vi "Warranty Gas Rack Main (FPGA).vi"() -> ()   [LabVIEW 2013]
uses:
  TypeDef/FPGADataCluster.ctl
  <vilib>/Platform/TimedLoop/XDataNode/timing_clust.ctl
  <vilib>/Platform/TimedLoop/XDataNode/nitl_modes.ctl
  <vilib>/Platform/TimedLoop/XDataNode/wakeup.ctl
  <vilib>/rvi/FXPMathLib/basic elements/FxpIntAccumulator/subVIs/nifxpmath_IntAccumulator_SimConfig.ctl
  <vilib>/rvi/FXPMathLib/FxpSqrt/subVIs/nifxpmath_Sqrt_SimConfig.ctl
  <vilib>/fxp/LVFixedPointOverflowPolicyTypeDef.ctl
  <vilib>/rvi/Emulation/niFpgaSctlEmulationGetInTimedLoop.vi
  <vilib>/rvi/Emulation/niFpgaEmulationReportErrorSimple.vi
  <vilib>/rvi/Emulation/niFpgaGetClockAttributes.vi
  <vilib>/rvi/eio/common/nirviEmuTemplateMethod_errors.vi
  <vilib>/rvi/Analysis/common/codeGenErrors/XNode/niFpgaXNodeCodeGenErrorHandle.vi
  <vilib>/rvi/Emulation/niFpgaCriticalErrorInLSC.vi
  <vilib>/rvi/FXPMathLib/basic elements/FxpIntAccumulator/simVIs/DllFxpIntAccumulator_sub.vi
  <vilib>/rvi/interface/RandomDataEmulation/nirviRandomDataFPGAFIFO.vi
  <vilib>/rvi/interface/RandomDataEmulation/niFpgaRandomDataHandleErrors.vi
  <vilib>/rvi/FXPMathLib/FxpSqrt/simVIs/DllSqrtTemp_sub.vi
  <vilib>/rvi/FXPMathLib/FxpSub/XNode/nifxpmath_Sub.xnode
  <vilib>/eio/EIONode/EIONode.xnode
  <vilib>/rvi/Analysis/measure/mean-var-std/XNode/niFpgaMean-Var-Std.xnode
  <vilib>/Platform/TimedLoop/XDataNode/XDataNode.xnode
  <vilib>/rvi/FXPMathLib/basic elements/FxpIntAccumulator/XNode/nifxpmath_IntAccumulator.xnode
  <vilib>/rvi/FXPMathLib/FxpMul/XNode/nifxpmath_Multiplier.xnode
  <vilib>/rvi/DataTransferAndStorage/Container/XNode/niFpgaContainer.xnode
  <vilib>/rvi/interface/RandomDataEmulation/nirviRandomDataFpgaReadWriteTemplate.vi
  <vilib>/rvi/Analysis/measure/butterworth/XNode/niFpgaButterworthFilter.xnode
  <vilib>/rvi/Analysis/measure/dc-rms/XNode/niFpgaDC-RMS.xnode
  <vilib>/rvi/FXPMathLib/FxpSqrt/XNode/nifxpmath_Sqrt.xnode
  <vilib>/Platform/TimedLoop/XDataNode/XDNodeRunTimeDep.lvlib
  <vilib>/rvi/FXPMathLib/sim/FxpSim.dll
panel:
  out "Version":u8=1
  in  "NeedleValve":bool
  in  "CtCuttoff":fxp<+,24,5>
  in  "Brushed Speed":bool
  in  "StableTrigger":fxp<+/-,20,5>
  in  "Count 2(uS)":u32=20
  out "AI3":fxp<+/-,24,5>
  out "AI7":fxp<+/-,24,5>
  out "AI6":fxp<+/-,24,5>
  out "AI4":fxp<+/-,24,5>
  out "AI2":fxp<+/-,24,5>
  out "AI1":fxp<+/-,24,5>
  out "AI0":fxp<+/-,24,5>
  out "Actual Loop Time 2":u32
  out "Actual Loop Time":u32
  in  "Count 1(uS)":u32=100
  in  "Hysteresis":fxp<+,24,5>
  out "DataCluster":T1 {"Speed" format="%#_6f"; "Controller Voltage" format="%#_6f"; "Controller Current" format="%#_6f"; "Temperature" format="%#_6f"}
  in  "PWM Period (ticks)":u32
  in  "PWM Duty":i32
  in  "Deadhead":bool
  in  "PSenable":bool
  in  "PresCtrl":fxp<+/-,20,5>
  in  "VoltCtrl":fxp<+/-,20,5>
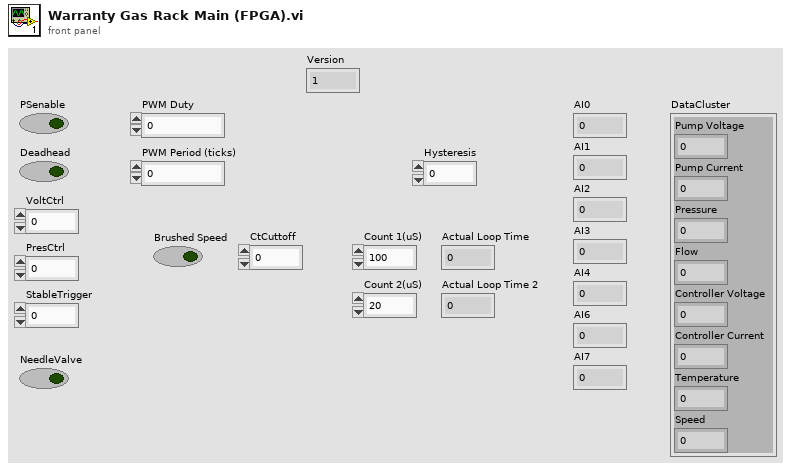
[diagram p1: front panel]
types:
  T1 = typedef "FPGADataCluster.ctl" = cluster{"Pump Voltage":fxp<+/-,25,15>, "Pump Current":fxp<+/-,25,15>, "Pressure":fxp<+/-,25,15>, "Flow":fxp<+/-,25,15>, "Controller Voltage":fxp<+/-,25,15>, "Controller Current":fxp<+/-,25,15>, "Temperature":fxp<+/-,25,15>, "Speed":fxp<+/-,25,15>}
  T2 = typedef "XDNodeRunTimeDep.lvlib/timing_clust.ctl" = cluster{"Expected End [f-1]":u64, "Actual End [f-1]":u64, "Finished Late? [f-1]":bool, "Expected End [i-1]":u64, "Actual End [i-1]":u64, "Finished Late? [i-1]":bool, "Expected Start [i]":u64, "Actual Start [i]":u64, "Expected Start [f]":u64, "Actual Start [f]":u64, "Source Name":string, "Structure Name":string, "Period":i64, "Deadline":i64, "Offset":i64, "Start":i64, "Priority":i32, "Timeout":i32, "Mode":T3, "Wakeup Reason":T4, "Error":errorcluster, "Source Type":string, "Secondary Source Type":string, "Global End Time":u64, "Global Start Time":u64, "Frame Duration":u64, "Iteration Duration":u64, "Assigned CPU":i32, "I/O Scan Engine Mode":u32}
  T3 = typedef "XDNodeRunTimeDep.lvlib/nitl_modes.ctl" = enum32{"No Change", "Process missed periods, maintain original phase", "Discard missed periods, maintain original phase", "Process missed periods, ignore original phase", "Discard missed periods, ignore original phase"}
  T4 = typedef "XDNodeRunTimeDep.lvlib/wakeup.ctl" = enum32{"Normal", "Aborted", "Asynchronous wakeup", "Timing source error", "Timed loop error", "Timeout"}
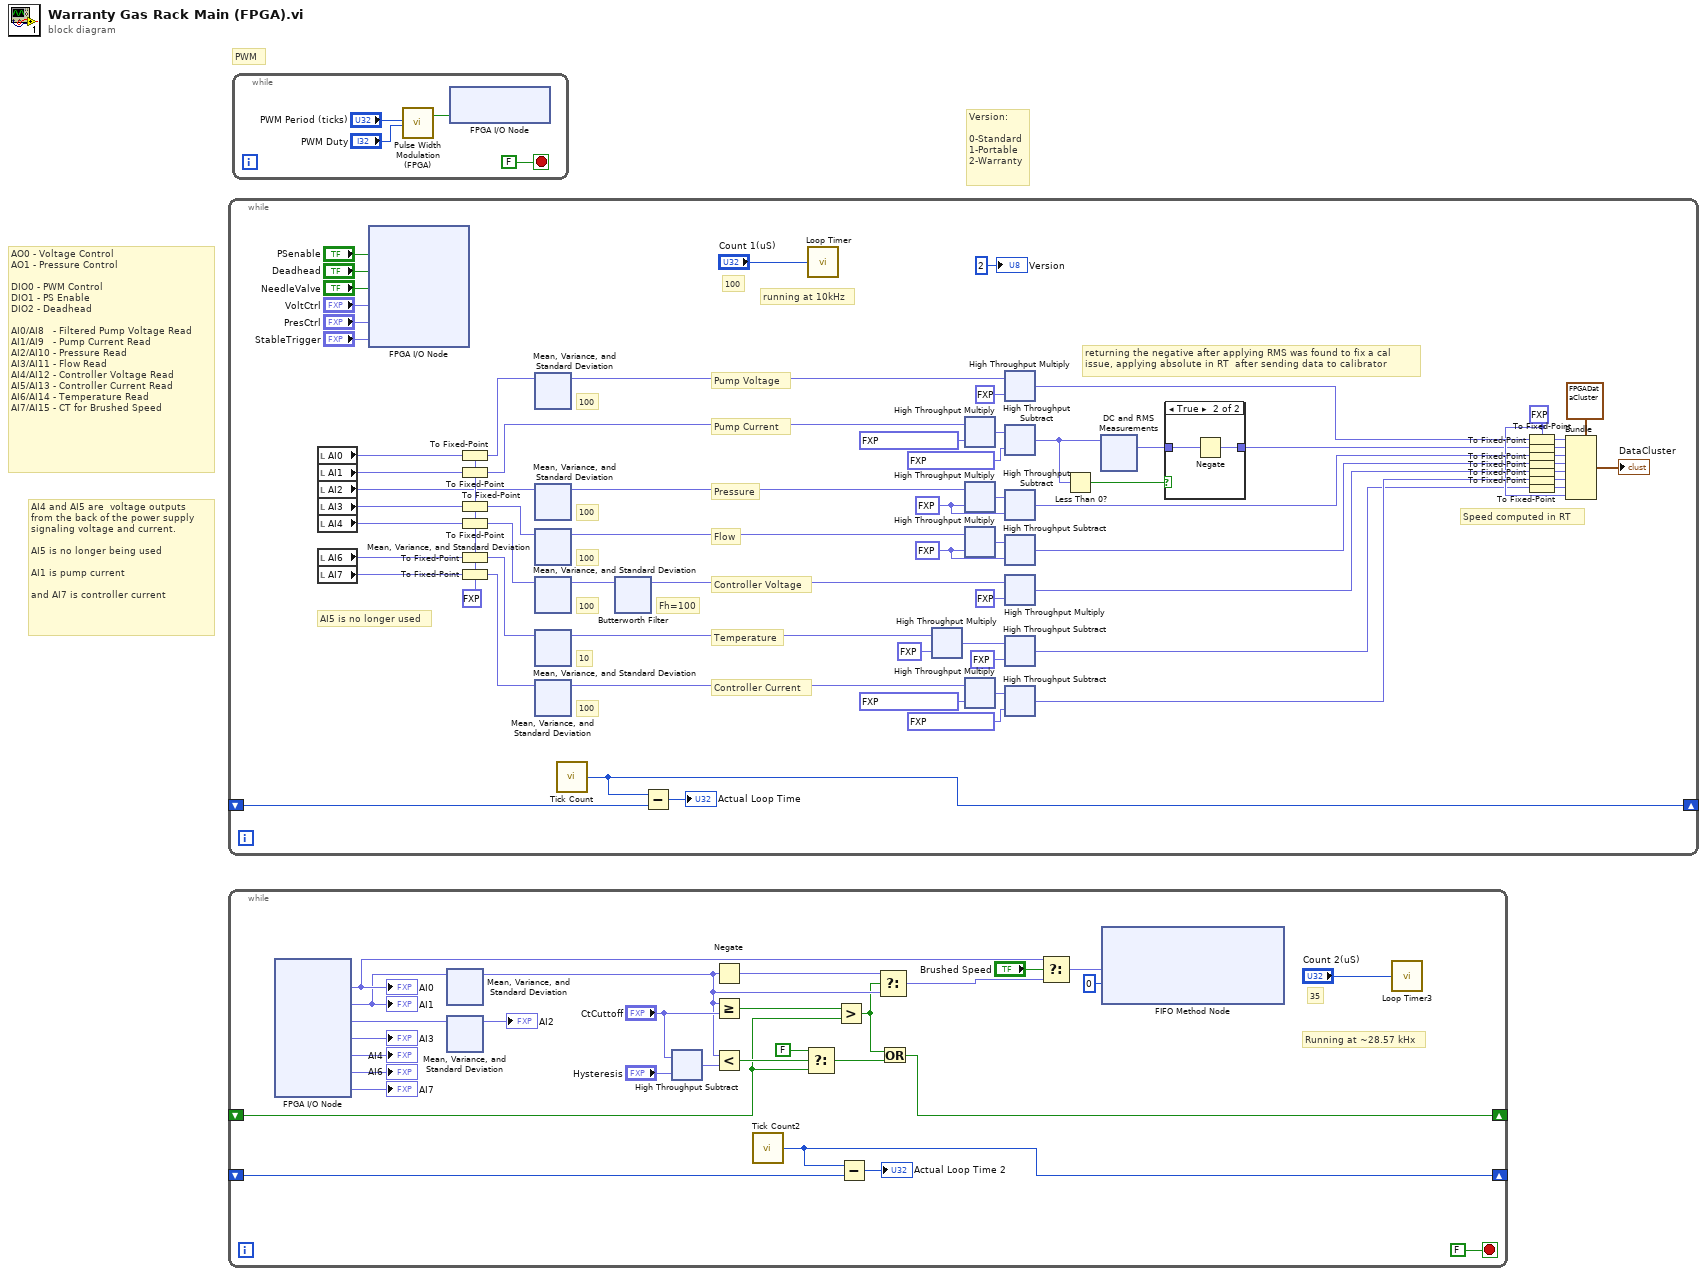
[diagram p0: block diagram]
diagram:
  # "Version:\n\n0-Standard\n1-Portable\n2-Warranty"
  # "PWM"
  # "AI4 and AI5 are  voltage outputs\nfrom the back of the power supply\nsignaling voltage and current.\n\nAI5 is no longer being used\n\nAI1 is pump current\n\nand AI7 is controller current"
  # "AO0 - Voltage Control\nAO1 - Pressure Control\n\nDIO0 - PWM Control\nDIO1 - PS Enable\nDIO2 - Deadhead\n\nAI0/AI8   - Filtered Pump Voltage Read\nAI1/AI9   - Pump Current Read\nAI2/AI10 - Pressure Read\nAI3/AI11 - Flow Read\nAI4/AI12 - Controller Voltage Read\nAI5/AI13 - Controller Current Read\nAI6/AI14 - Temperature Read\nAI7/AI15 - CT for Brushed Speed"
  n1 = while {
    shift-right: [w33] -> _
    shift-left: _ -> [w32]
    stop <- FALSE stop-if-true
    w20 = fxp<+,9,9> 258.0 ("y")
    w43 = fxp<+,24,5> 0.0 ("AI4")
    w11 = fxp<+/-,25,15> 0.0 ("Element")
    w4 = fxp<+,8,8> 170.0 ("y")
    # "Fh=100"
    # "10"
    # "100"
    # "100"
    # "100"
    # "100"
    # "100"
    # "Temperature"
    # "Controller Current"
    # "Controller Voltage"
    # "Flow"
    # "Pressure"
    # "Pump Current"
    # "Pump Voltage"
    # "100"
    # "Speed computed in RT"
    # "returning the negative after applying RMS was found to fix a cal\nissue, applying absolute in RT  after sending data to calibrator"
    # "AI5 is no longer used"
    # "running at 10kHz"
    n2 = local read "AI0"() -> (w31:fxp<+/-,24,5>)
    n3 = local read "AI1"() -> (w30:fxp<+/-,24,5>)
    n4 = local read "AI2"() -> (w15:fxp<+/-,24,5>)
    n5 = local read "AI3"() -> (w28:fxp<+/-,24,5>)
    n6 = local read "AI4"() -> (w27:fxp<+/-,24,5>)
    n7 = local read "AI6"() -> (w26:fxp<+/-,24,5>)
    n8 = local read "AI7"() -> (w29:fxp<+/-,24,5>)
    n9 = xnode "FPGA I/O Node"("RMC/DIO1"="PSenable", "RMC/DIO2"="Deadhead", "RMC/DIO3"="NeedleValve", "AO0"="VoltCtrl", "AO1"="PresCtrl", "AO2"="StableTrigger") -> ()  [unwired: 6 in, 6 out]
    n10 = To Fixed-Point(fixed-point type=w43, number=w31) -> (fixed-point=w36:fxp<+,24,5>)
    n11 = To Fixed-Point(fixed-point type=w43, number=w30) -> (fixed-point=w10:fxp<+,24,5>)
    n12 = To Fixed-Point(fixed-point type=w43, number=w28) -> (fixed-point=w42:fxp<+,24,5>)
    n13 = To Fixed-Point(fixed-point type=w43, number=w27) -> (fixed-point=w41:fxp<+,24,5>)
    n14 = To Fixed-Point(fixed-point type=w43, number=w26) -> (fixed-point=w35:fxp<+,24,5>)
    n15 = To Fixed-Point(fixed-point type=w43, number=w29) -> (fixed-point=w17:fxp<+,24,5>)
    n16 = xnode "Mean, Variance, and Standard Deviation"("input data"=w36) -> ("mean"=w40:fxp<+,24,5>)  [unwired: 1 in, 1 out]
    n17 = xnode "Mean, Variance, and Standard Deviation"("input data"=w15) -> ("mean"=w14:fxp<+/-,24,5>)  [unwired: 1 in, 1 out]
    n18 = xnode "Mean, Variance, and Standard Deviation"("input data"=w42) -> ("mean"=w39:fxp<+,24,5>)  [unwired: 1 in, 1 out]
    n19 = xnode "Mean, Variance, and Standard Deviation"("input data"=w41) -> ("mean"=w13:fxp<+,24,5>)  [unwired: 1 in, 1 out]
    n20 = xnode "Mean, Variance, and Standard Deviation"("input data"=w35) -> ("mean"=w7:fxp<+,24,5>)  [unwired: 1 in, 1 out]
    n21 = xnode "Mean, Variance, and Standard Deviation"("input data"=w17) -> ("mean"=w16:fxp<+,24,5>)  [unwired: 1 in, 1 out]
    n22 = call "Tick Count"() -> ("Tick Count(uSec)"=w33:u32)
    n23 = xnode "Butterworth Filter"("input data"=w13) -> ("output data"=w12:fxp<+/-,29,10>)  [unwired: 2 in]
    n24 = Subtract(x=w33, y=w32) -> (x-y=→"Actual Loop Time":u32)
    n25 = call "Loop Timer"("Count(uSec)"="Count 1(uS)") -> ()  [unwired: 1 out]
    n26 = xnode ("High Throughput Multiply")("x"=w7, "y"=fxp<+/-,9,9> 145.0) -> ("x*y"=w6:fxp<+/-,25,15>)
    n27 = xnode ("High Throughput Multiply")("x"=w10, "y"=fxp<+/-,20,7> 24.0384521484375 ("Volt")) -> ("x*y"=w66:fxp<+/-,44,12>)
    n28 = xnode ("High Throughput Multiply")("x"=w14, "y"=w20) -> ("x*y"=w22:fxp<+/-,33,14>)
    n29 = xnode ("High Throughput Multiply")("x"=w39, "y"=w4) -> ("x*y"=w5:fxp<+/-,25,15>)
    n30 = xnode ("High Throughput Multiply")("x"=w16, "y"=fxp<+/-,20,7> 24.0384521484375 ("Volt")) -> ("x*y"=w37:fxp<+/-,44,12>)
    n31 = xnode ("High Throughput Multiply")("x"=w40, "y"=fxp<+/-,24,5> 11.0) -> ("x*y"=w48:fxp<+/-,25,15>)
    n32 = xnode "High Throughput Subtract"("x"=w66, "y"=fxp<+/-,20,7> 60.09619140625 ("Volt")) -> ("x-y"=w19:fxp<+/-,25,15>)
    n33 = xnode "High Throughput Subtract"("x"=w22, "y"=w20) -> ("x-y"=w21:fxp<+/-,34,15>)
    n34 = xnode "High Throughput Subtract"("x"=w5, "y"=w4) -> ("x-y"=w3:fxp<+/-,26,16>)
    n35 = xnode ("High Throughput Multiply")("x"=w12, "y"=fxp<+,8,8> 11.0) -> ("x*y"=w47:fxp<+/-,25,15>)
    n36 = xnode "High Throughput Subtract"("x"=w6, "y"=fxp<+/-,8,8> 100.0) -> ("x-y"=w8:fxp<+/-,21,10>)
    n37 = xnode "High Throughput Subtract"("x"=w37, "y"=fxp<+/-,20,7> 60.09619140625 ("Volt")) -> ("x-y"=w18:fxp<+/-,25,15>)
    n38 = Less Than 0?(x=w19) -> (x < 0?=w24:bool)
    n39 = xnode "DC and RMS Measurements"("input data"=w19) -> ("RMS"=w23:fxp<+,25,15>)  [unwired: 1 in, 1 out]
    n40 = case shown="True" w24 {
      tunnel: w23 -> [w229 w231]
      tunnel: [w229 w230] -> w2
      frame False {
      }
      frame True {
        n41 = Negate(x=w231) -> (-x=w230:fxp<+/-,26,16>)
      }
    }
    n42 = To Fixed-Point(fixed-point type=w11, number=w48) -> (fixed-point=w55:fxp<+/-,25,15>)
    n43 = To Fixed-Point(fixed-point type=w11, number=w2) -> (fixed-point=w56:fxp<+/-,25,15>)
    n44 = To Fixed-Point(fixed-point type=w11, number=w21) -> (fixed-point=w57:fxp<+/-,25,15>)
    n45 = To Fixed-Point(fixed-point type=w11, number=w3) -> (fixed-point=w58:fxp<+/-,25,15>)
    n46 = To Fixed-Point(fixed-point type=w11, number=w47) -> (fixed-point=w59:fxp<+/-,25,15>)
    n47 = To Fixed-Point(fixed-point type=w11, number=w18) -> (fixed-point=w50:fxp<+/-,25,15>)
    n48 = To Fixed-Point(fixed-point type=w11, number=w8) -> (fixed-point=w51:fxp<+/-,25,15>)
    n49 = Bundle(cluster=T1 {"Pump Voltage"=0.0, "Pump Current"=0.0, "Pressure"=0.0, "Flow"=0.0, "Controller Voltage"=0.0, "Controller Current"=0.0, "Temperature"=0.0, "Speed"=0.0} ("DataCluster"), "Pump Voltage"=w55, "Pump Current"=w56, "Pressure"=w57, "Flow"=w58, "Controller Voltage"=w59, "Controller Current"=w50, "Temperature"=w51, "Speed"=w11) -> (→"DataCluster":T1)
    "Version" <- u8 2
  }
  n50 = while {
    shift-right: [w669] -> _
    shift-left: _ -> [w670]
    shift-right: [w646] -> _
    shift-left: _ -> [w650]
    stop <- FALSE stop-if-true
    # "Running at ~28.57 kHx"
    # "35"
    n51 = xnode "FPGA I/O Node"() -> ("AI0"=w659:fxp<+/-,24,5>, "AI1"=w657:fxp<+/-,24,5>, "AI2"=w645:fxp<+/-,24,5>, "AI3"=→"AI3":fxp<+/-,24,5>, "AI4"=→"AI4":fxp<+/-,24,5>, "AI6"=→"AI6":fxp<+/-,24,5>, "AI7"=→"AI7":fxp<+/-,24,5>)  [unwired: 7 in, 7 out]
    "AI0" <- w659
    "AI1" <- w657
    n52 = xnode "Mean, Variance, and Standard Deviation"("input data"=w657) -> ("mean"=w653:fxp<+/-,24,5>)  [unwired: 1 in, 1 out]
    n53 = xnode "Mean, Variance, and Standard Deviation"("input data"=w645) -> ("mean"=→"AI2":fxp<+/-,24,5>)  [unwired: 1 in, 1 out]
    n54 = xnode "High Throughput Subtract"("x"="CtCuttoff", "y"="Hysteresis") -> ("x-y"=w652:fxp<+/-,25,15>)
    n55 = Negate(x=w653) -> (-x=w662:fxp<+/-,25,6>)
    n56 = Greater Or Equal?(x=w653, y="CtCuttoff") -> (x >= y?=w658:bool)
    n57 = Less?(x=w653, y=w652) -> (x < y?=w651:bool)
    n58 = call "Tick Count2"() -> ("Tick Count(uSec)"=w669:u32)
    n59 = Select(t=FALSE, s=w651, f=w650) -> (s? t:f=w648:bool)
    n60 = Greater?(x=w658, y=w650) -> (0:w647:bool)
    n61 = Subtract(x=w669, y=w670) -> (x-y=→"Actual Loop Time 2":u32)
    n62 = Select(t=w662, s=w647, f=w653) -> (s? t:f=w660:fxp<+/-,25,6>)
    n63 = Or(x=w647, y=w648) -> (x .or. y?=w646:bool)
    n64 = Select(t=w659, s="Brushed Speed", f=w660) -> (s? t:f=w656:fxp<+/-,25,6>)
    n65 = xnode ("FIFO Method Node")("Element"=w656, "Timeout"=0) -> ()  [unwired: 1 in, 2 out]
    n66 = call "Loop Timer3"("Count(uSec)"="Count 2(uS)") -> ()  [unwired: 1 out]
  }
  n67 = while {
    stop <- FALSE stop-if-true
    n68 = call "Pulse Width Modulation (FPGA).vi"("PWM Period (Ticks)"="PWM Period (ticks)", "PWM Duty Cycle (Ticks)"="PWM Duty") -> ("PWM DO"=w828:bool)  [unwired: 14 in, 3 out]
    n69 = xnode "FPGA I/O Node"("RMC/DIO0"=w828) -> ()  [unwired: 1 in, 1 out]
  }
